vi "disconnect.vi"(8 "error in (no error)":errorcluster, 11 "AlCS in":refnum<class "AlCS.lvclass">) -> (0 "error out":errorcluster, 3 "AlCS out":refnum<class "AlCS.lvclass">)   [LabVIEW 2016, in "AlCS.lvclass"]
uses:
  AlCS.lvclass
  AlCS.lvclass/AlCS.ctl
  ts_labview_tcp/TCPClient/TCPClient.lvclass
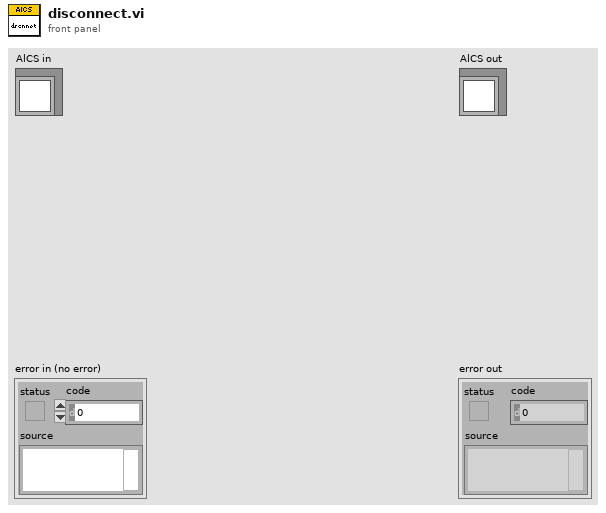
[diagram p1: front panel]
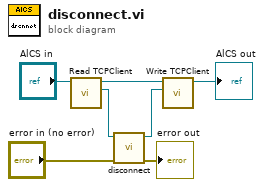
[diagram p0: block diagram]
diagram:
  n1 = call "Read TCPClient.vi"("AlCS in"="AlCS in") -> ("TCPClient.lvclass"=w3:refnum<class "TCPClient.lvclass">, "AlCS out"=w7:refnum<class "AlCS.lvclass">)  [unwired: 8 in, 1 out]
  n2 = call-dynamic "disconnect.vi"("error in (no error)"="error in (no error)", "TCPClient in"=w3) -> ("error out"=→"error out":errorcluster, "TCPClient out"=w4:refnum<class "TCPClient.lvclass">)  [unwired: 8 in]
  n3 = call "Write TCPClient.vi"("TCPClient.lvclass"=w4, "AlCS in"=w7) -> ("AlCS out"=→"AlCS out":refnum<class "AlCS.lvclass">)  [unwired: 8 in, 1 out]
